vi "PH_BeamlineController.panel.vi"() -> ()   [LabVIEW 2014, in "PH_BeamlineController.lvlib"]
uses:
  PH_BeamlineController.lvlib
  PH_Beamline_Chief/PH_Beamline_Chief.Section.ctl
  PH_BeamlineInformation/PH_BeamlineInformation.Powermeter.ctl
  PH_BeamlineInformation/PH_BeamlineInformation.Efficiency.ctl
  PH_SystemInformation/PH_SystemInformation.GUI Refs.ctl
  PH_BeamlineController.Source Attributes.ctl
  PH_BeamlineController.Sources.ctl
  PH_BeamlineController.Target Attributes.ctl
  PH_BeamlineController.Targets.ctl
  PH_BeamlineController.PA DP Target Attributes.ctl
  PH_BeamlineController.PA DP Targets.ctl
  PH_BeamlineController.special GUI Refs.ctl
  PH_BeamlineInformation/PH_BeamlineInformation.GUI Ref.ctl
  PH_Common/PH_Common.lvlib
  PH_Beamline_Chief/PH_Beamline_Chief.lvlib
  PH_BeamlineInformation/PH_BeamlineInformation.lvlib
  PH_Synchrolock_Watch/PH_Synchrolock_Watch.lvlib
  PH_BackreflectionMeas/PH_BackreflectionMeas.lvlib
  CSCore/CSSystem/CSSystemLib/CSSystemLib.lvlib
  PH_SystemInformation/PH_SystemInformation.lvlib
  PH_Class/PH_Class.lvlib
panel:
  in  "Accept":bool
  out "PIL_Exp4_ShutterDisabled":u32(colorbox)=6618880 caption="Z6 enabled"
  out "Emergency Off":u32(colorbox)=16711680
  out "Laser enabled":u32(colorbox)=6618880
  out "PHELIX_Beamline_MA_LB_BL_Status 2":u32(colorbox)
  in  "PA-Backreflection-Meas":bool caption="B"
  in  "fs_Synchrolock_Watch":bool caption="S"
  out "PHELIX_Beamline_PA_before_Bypass_BL_Status":u32(colorbox)
  out "PHELIX_Beamline_PA_BL_Status":u32(colorbox)
  out "PHELIX_Beamline_LB_TB2_BL_Status":u32(colorbox)
  out "PHELIX_Beamline_Z6_BL_Status":u32(colorbox)
  out "PHELIX_Beamline_LL_BL_Status":u32(colorbox)
  out "PHELIX_Beamline_MA_Exit_BL_Status":u32(colorbox)
  out "PHELIX_Beamline_PA_Exit_BL_Status":u32(colorbox)
  out "PHELIX_Beamline_PA_Input_BL_Status":u32(colorbox)
  out "PHELIX_Beamline_PA_UnDelay_BL_Status":u32(colorbox)
  out "PHELIX_Beamline_fs_YLF_BL_Status":u32(colorbox)
  out "PHELIX_Beamline_YLF_BL_Status 2":u32(colorbox)
  out "PHELIX_Beamline_ns_BL_Status 2":u32(colorbox)
  out "PHELIX_Beamline_PA_Bypass_BL_Status 3":u32(colorbox)
  out "PHELIX_Beamline_PA_Bypass_BL_Status 2":u32(colorbox)
  out "PHELIX_Beamline_PA_Bypass_BL_Status 1":u32(colorbox)
  out "PHELIX_Beamline_PA_Delay_BL_Status 3":u32(colorbox)
  out "PHELIX_Beamline_PA_Input_BL_Status 1":u32(colorbox)
  out "PHELIX_Beamline_PA_Delay_BL_Status 2":u32(colorbox)
  out "PHELIX_Beamline_MA_Z6_BL_Status":u32(colorbox)
  out "PHELIX_Beamline_MA_LB_BL_Status 1":u32(colorbox)
  out "PHELIX_Beamline_MA_LB_BL_Status":u32(colorbox)
  out "PHELIX_Beamline_YLF_BL_Status 1":u32(colorbox)
  out "PHELIX_Beamline_fs_BL_Status":u32(colorbox)
  out "PHELIX_Beamline_ns_BL_Status 1":u32(colorbox)
  out "PHELIX_Beamline_PA_LL_BL_Status 2":u32(colorbox)
  out "PHELIX_Beamline_PA_LL_BL_Status 1":u32(colorbox)
  out "PHELIX_Beamline_PA_MA_BL_Status":u32(colorbox)
  in  "Delete":bool
  out "error out":errorcluster
  in  "error in (no error)":errorcluster
  in  "object ref":refnum<vi>
  out "PHELIX_Beamline_LB_TB3_BL_Status":u32(colorbox)
  in  "Experiment Z6":bool caption="Z6"
  in  "Experiment Laserlabor":bool caption="LL"
  in  "Calorimeter":bool caption="MA"
  in  "PreAmp":bool caption="PA"
  in  "ns-Frontend":bool caption="ns"
  in  "fs-Frontend":bool caption="fs"
  in  "YLF":bool
  in  "Dump Laserbay":bool
  in  "Dump Z6":bool
  in  "Dump Laserlabor":bool
  in  "Dump PA Undelayed":bool
  in  "Dump PA Delayed":bool
  out "Experiment_VacuumControl_Experiment":bool caption="V"
  in  "Experiment Laserbay":bool caption="LB"
  # "PCS"
  # "3.40"
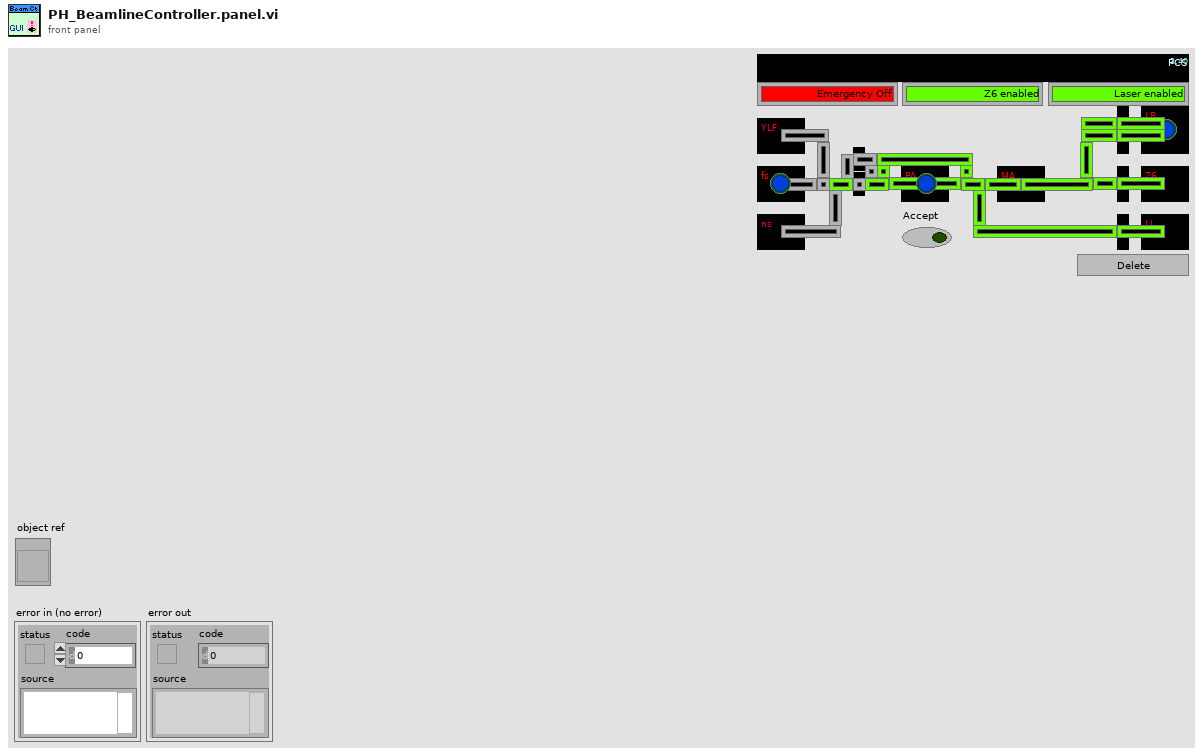
[diagram p1: front panel]
types:
  T1 = typedef "PH_BeamlineController.lvlib/PH_BeamlineController.Source Attributes.ctl" = cluster{"Name":T2, "GUI Ref":refnum<vi>, "Current State":bool, "Wanted State":bool}
  T2 = typedef "PH_BeamlineController.lvlib/PH_BeamlineController.Sources.ctl" = enum16{"None", "YLF", "fs-Frontend", "ns-Frontend", "YLF and ns-Frontend", "fs- and ns-Frontend"}
  T3 = typedef "PH_BeamlineController.lvlib/PH_BeamlineController.PA DP Target Attributes.ctl" = cluster{"Name":T4, "GUI Ref":refnum<vi>, "Current State":bool, "Wanted State":bool, "Enabled":bool}
  T4 = typedef "PH_BeamlineController.lvlib/PH_BeamlineController.PA DP Targets.ctl" = enum16{"None", "Dump PA Delayed Beam", "Dump PA Undelayed Beam", "Dumps PA Delayed and Undelayed Beam"}
  T5 = typedef "PH_BeamlineController.lvlib/PH_BeamlineController.Target Attributes.ctl" = cluster{"Name":T6, "GUI Ref":refnum<vi>, "Current State":bool, "Wanted State":bool, "Enabled":bool}
  T6 = typedef "PH_BeamlineController.lvlib/PH_BeamlineController.Targets.ctl" = enum16{"None", "PreAmp", "Dump Exp Laserlab", "Exp Laserlab", "Calorimeter", "Dump Exp Laserbay", "Exp Laserbay", "Dump Exp Z6", "Exp Z6"}
  T7 = typedef "PH_BeamlineController.lvlib/PH_BeamlineController.special GUI Refs.ctl" = cluster{"PA-Backreflection-Meas":refnum<vi>, "fs_Synchrolock_Watch":refnum<vi>}
  T8 = typedef "PH_BeamlineInformation.lvlib/PH_BeamlineInformation.GUI Ref.ctl" = cluster{"BL Elements":cluster{"GUI Ref":refnum<vi>, "Beamline Section":T9}[], "Powermeters":T10, "Efficiency GUI Refs":T11, "Head GUI Refs":cluster{"PA - 19 - 1":cluster{"in Use":refnum<vi>, "voltage":refnum<vi>}, "PA - 19 - 2":cluster{"in Use":refnum<vi>, "voltage":refnum<vi>}, "PA - 45":cluster{"in Use":refnum<vi>, "voltage":refnum<vi>}, "PA - 45 - DP":cluster{"in Use":refnum<vi>, "voltage":refnum<vi>}, "MA - 1":cluster{"in Use":refnum<vi>, "voltage":refnum<vi>}, "MA - 2":cluster{"in Use":refnum<vi>, "voltage":refnum<vi>}, "MA - 3":cluster{"in Use":refnum<vi>, "voltage":refnum<vi>}, "MA - 4":cluster{"in Use":refnum<vi>, "voltage":refnum<vi>}, "MA - 5":cluster{"in Use":refnum<vi>, "voltage":refnum<vi>}, "MA - FR":cluster{"in Use":refnum<vi>, "voltage":refnum<vi>}}, "System Information GUI Refs":T12}
  T9 = typedef "PH_Beamline_Chief.lvlib/PH_Beamline_Chief.Section.ctl" = enum16{"None", "YLF", "fs", "fs-YLF", "ns", "PA-Input", "PA-Undelay", "PA-Delay", "PA-before-Bypass", "PA", "PA-Bypass", "PA-Exit", "PA-LL", "LL", "PA-MA", "MA-Exit", "MA-Z6", "Z6", "MA-LB", "LB-TB2", "LB-TB3"}
  T10 = typedef "PH_BeamlineInformation.lvlib/PH_BeamlineInformation.Powermeter.ctl" = cluster{"ns FE":cluster{"GUI Ref":refnum<vi>, "Value":dbl}, "fs FE":cluster{"GUI Ref":refnum<vi>, "Value":dbl}, "PA":cluster{"GUI Ref":refnum<vi>, "Value":dbl}, "MA":cluster{"GUI Ref":refnum<vi>, "Value":dbl}, "Z6 green":cluster{"GUI Ref":refnum<vi>, "Value":dbl}, "Z6 IR":cluster{"GUI Ref":refnum<vi>, "Value":dbl}, "Z6 COS":cluster{"GUI Ref":refnum<vi>, "Value":dbl}}
  T11 = typedef "PH_BeamlineInformation.lvlib/PH_BeamlineInformation.Efficiency.ctl" = cluster{"PA Gain":cluster{"GUI Ref":refnum<vi>, "Value":dbl}, "MA Gain":cluster{"GUI Ref":refnum<vi>, "Value":dbl}, "Z6 green Conversion":cluster{"GUI Ref":refnum<vi>, "Value":dbl}, "Z6 Comp Losses":cluster{"GUI Ref":refnum<vi>, "Value":dbl}}
  T12 = typedef "PH_SystemInformation.lvlib/PH_SystemInformation.GUI Refs.ctl" = cluster{"Laser":refnum<vi>, "PreAmp":refnum<vi>, "MainAmp":refnum<vi>, "Emergency Off":refnum<vi>, "Exp 1":refnum<vi>, "Exp 2":refnum<vi>, "Exp 3":refnum<vi>, "Exp 4":refnum<vi>, "Timing Mode GUI Ref":refnum<vi>}
  T13 = cluster{"Sources":T1[], "Side Targets":T3[], "Targets":T5[], "Experiment_VacuumControl_Experiment":refnum<vi>, "special GUI Refs":T7, "Beamline Information GUI Refs":T8}
  T14 = cluster{"PA - 19 - 1":cluster{"in Use":refnum<vi>, "voltage":refnum<vi>}, "PA - 19 - 2":cluster{"in Use":refnum<vi>, "voltage":refnum<vi>}, "PA - 45":cluster{"in Use":refnum<vi>, "voltage":refnum<vi>}, "PA - 45 - DP":cluster{"in Use":refnum<vi>, "voltage":refnum<vi>}, "MA - 1":cluster{"in Use":refnum<vi>, "voltage":refnum<vi>}, "MA - 2":cluster{"in Use":refnum<vi>, "voltage":refnum<vi>}, "MA - 3":cluster{"in Use":refnum<vi>, "voltage":refnum<vi>}, "MA - 4":cluster{"in Use":refnum<vi>, "voltage":refnum<vi>}, "MA - 5":cluster{"in Use":refnum<vi>, "voltage":refnum<vi>}, "MA - FR":cluster{"in Use":refnum<vi>, "voltage":refnum<vi>}}
  T15 = cluster{"GUI Ref":refnum<vi>, "Beamline Section":T9}
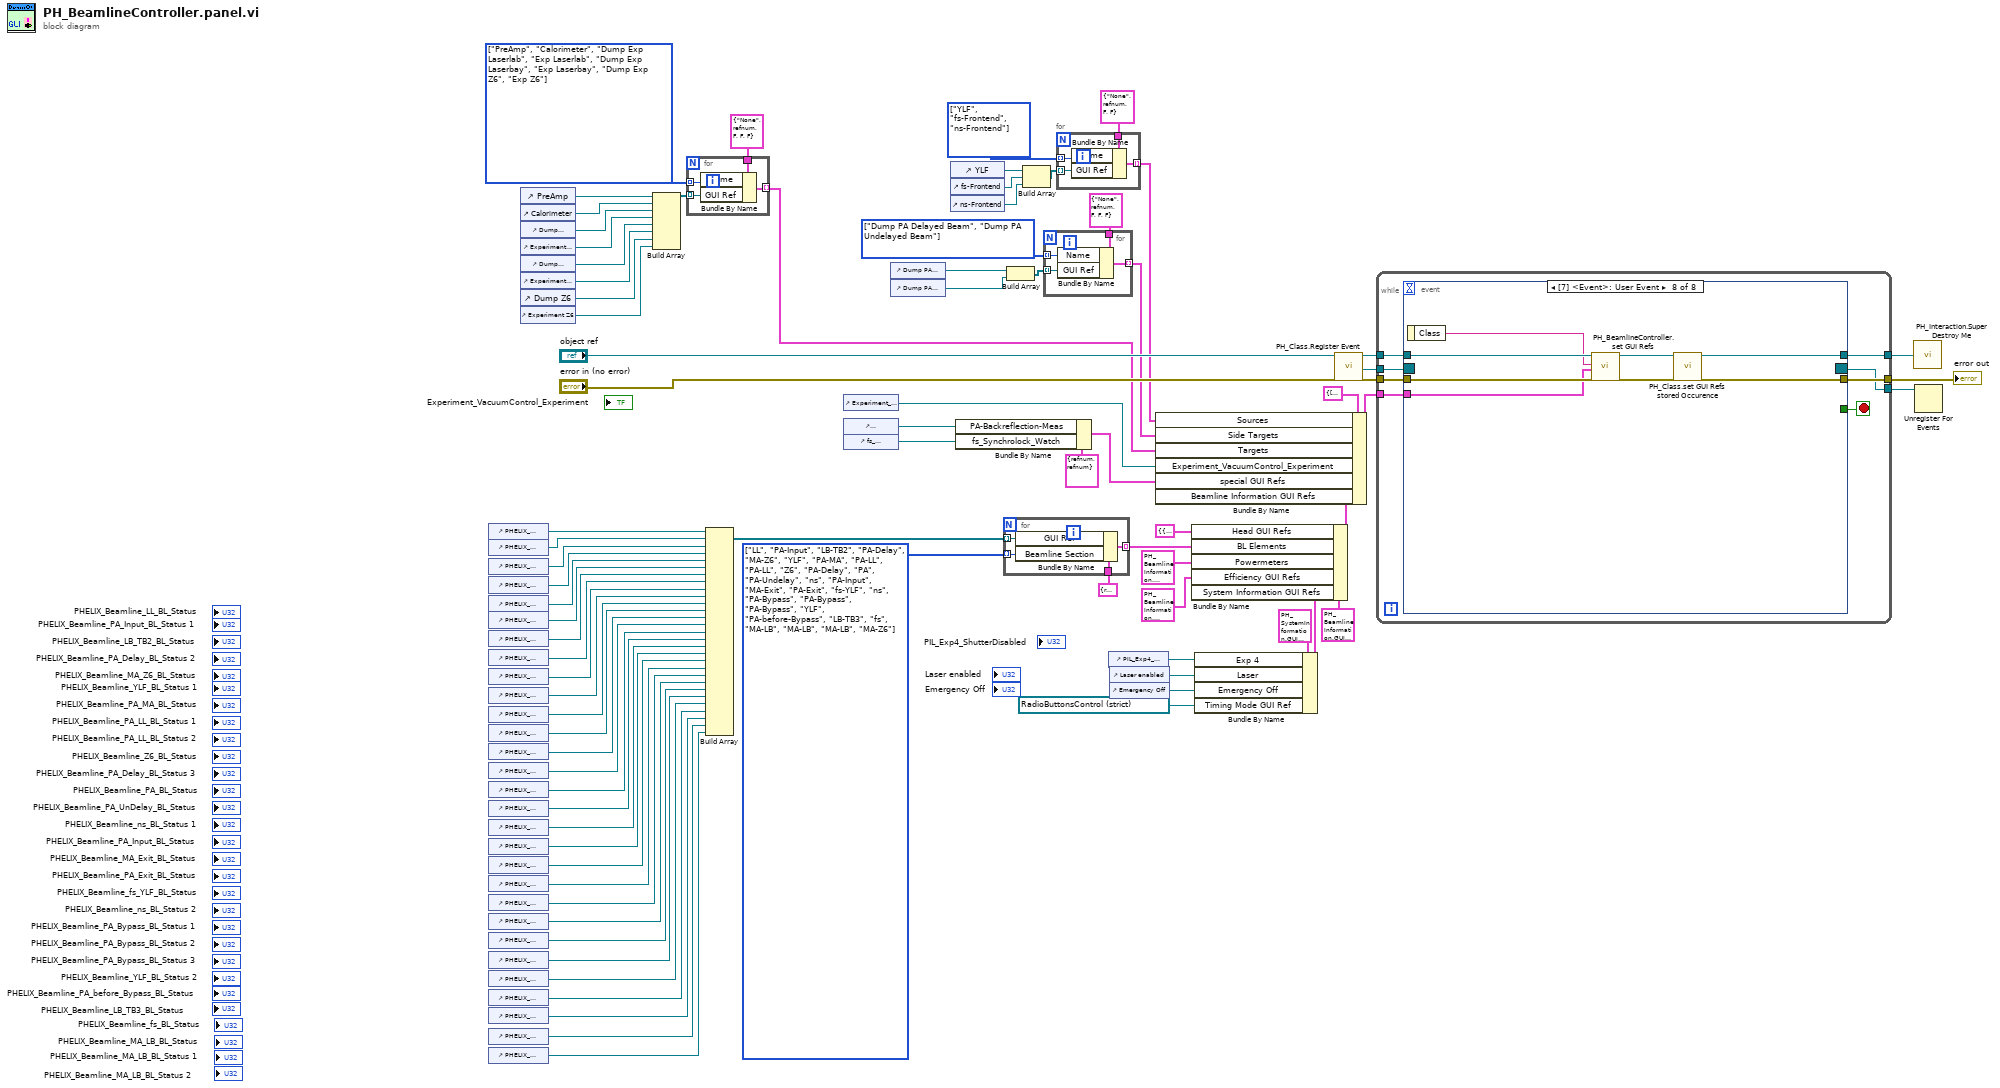
[diagram p0: block diagram]
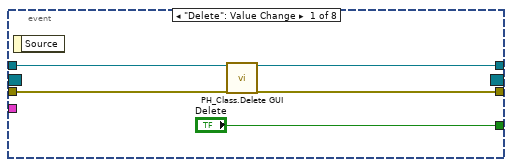
[diagram p2: hidden frame]
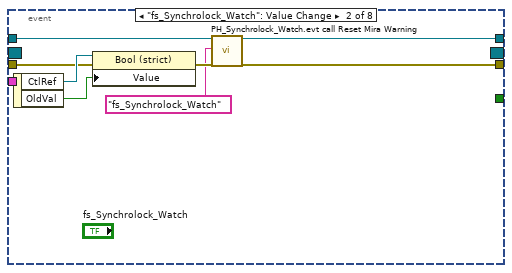
[diagram p3: hidden frame]
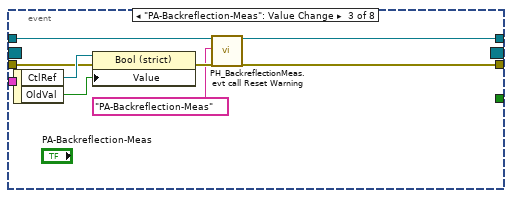
[diagram p4: hidden frame]
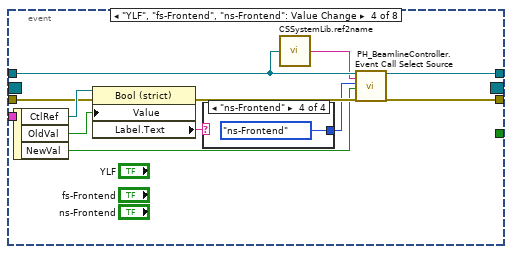
[diagram p5: hidden frame]
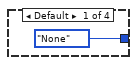
[diagram p6: hidden frame]
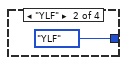
[diagram p7: hidden frame]
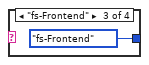
[diagram p8: hidden frame]
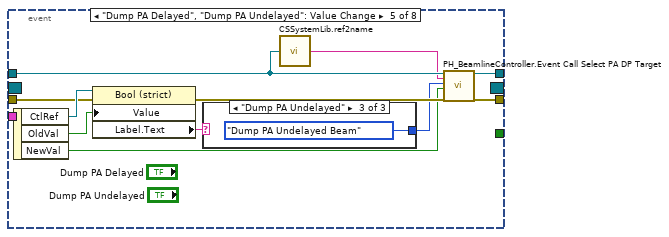
[diagram p9: hidden frame]
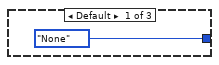
[diagram p10: hidden frame]
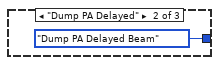
[diagram p11: hidden frame]
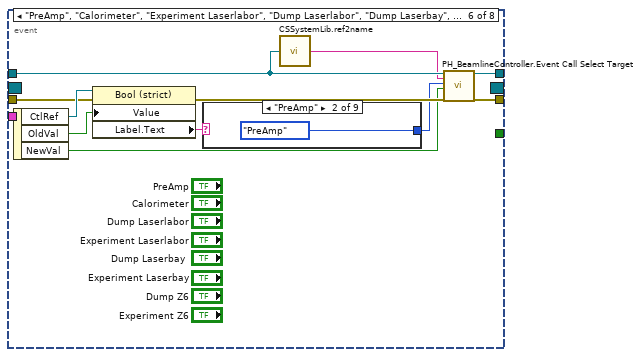
[diagram p12: hidden frame]
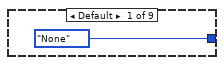
[diagram p13: hidden frame]
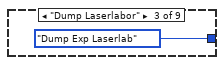
[diagram p14: hidden frame]
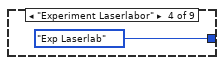
[diagram p15: hidden frame]
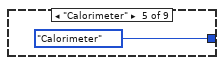
[diagram p16: hidden frame]
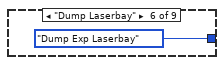
[diagram p17: hidden frame]
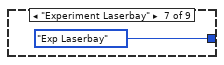
[diagram p18: hidden frame]
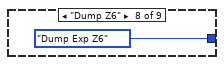
[diagram p19: hidden frame]
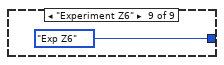
[diagram p20: hidden frame]
diagram:
  w17 = T4[] [enum."Dump PA Delayed Beam", enum."Dump PA Undelayed Beam"] items=["None", "Dump PA Delayed Beam", "Dump PA Undelayed Beam", "Dumps PA Delayed and Undelayed Beam"]
  w26 = T6[] [enum."PreAmp", enum."Calorimeter", enum."Dump Exp Laserlab", enum."Exp Laserlab", enum."Dump Exp Laserbay", enum."Exp Laserbay", enum."Dump Exp Z6", enum."Exp Z6"] items=["None", "PreAmp", "Dump Exp Laserlab", "Exp Laserlab", "Calorimeter", "Dump Exp Laserbay", "Exp Laserbay", "Dump Exp Z6", "Exp Z6"]
  w41 = T2[] [enum."YLF", enum."fs-Frontend", enum."ns-Frontend"] items=["None", "YLF", "fs-Frontend", "ns-Frontend", "YLF and ns-Frontend", "fs- and ns-Frontend"]
  w51 = T9[] [enum."LL", enum."PA-Input", enum."LB-TB2", enum."PA-Delay", enum."MA-Z6", enum."YLF", enum."PA-MA", enum."PA-LL", enum."PA-LL", enum."Z6", enum."PA-Delay", enum."PA", enum."PA-Undelay", enum."ns", enum."PA-Input", enum."MA-Exit", enum."PA-Exit", enum."fs-YLF", enum."ns", enum."PA-Bypass", enum."PA-Bypass", enum."PA-Bypass", enum."YLF", enum."PA-before-Bypass", enum."LB-TB3", enum."fs", enum."MA-LB", enum."MA-LB", enum."MA-LB", enum."MA-Z6"] items=["None", "YLF", "fs", "fs-YLF", "ns", "PA-Input", "PA-Undelay", "PA-Delay", "PA-before-Bypass", "PA", "PA-Bypass", "PA-Exit", "PA-LL", "LL", "PA-MA", "MA-Exit", "MA-Z6", "Z6", "MA-LB", "LB-TB2", "LB-TB3"]
  n1 = control-ref of="PHELIX_Beamline_LL_BL_Status"() -> (w82:refnum<vi>)
  n2 = control-ref of="PHELIX_Beamline_PA_Input_BL_Status 1"() -> (w81:refnum<vi>)
  n3 = control-ref of="PHELIX_Beamline_LB_TB2_BL_Status"() -> (w80:refnum<vi>)
  n4 = control-ref of="PHELIX_Beamline_PA_Delay_BL_Status 2"() -> (w79:refnum<vi>)
  n5 = control-ref of="PHELIX_Beamline_MA_Z6_BL_Status"() -> (w78:refnum<vi>)
  n6 = control-ref of="PHELIX_Beamline_YLF_BL_Status 1"() -> (w77:refnum<vi>)
  n7 = control-ref of="PHELIX_Beamline_PA_MA_BL_Status"() -> (w76:refnum<vi>)
  n8 = control-ref of="PHELIX_Beamline_PA_LL_BL_Status 1"() -> (w75:refnum<vi>)
  n9 = control-ref of="PHELIX_Beamline_PA_LL_BL_Status 2"() -> (w74:refnum<vi>)
  n10 = control-ref of="PHELIX_Beamline_Z6_BL_Status"() -> (w73:refnum<vi>)
  n11 = control-ref of="PHELIX_Beamline_PA_Delay_BL_Status 3"() -> (w72:refnum<vi>)
  n12 = control-ref of="PHELIX_Beamline_PA_BL_Status"() -> (w71:refnum<vi>)
  n13 = control-ref of="PHELIX_Beamline_PA_UnDelay_BL_Status"() -> (w70:refnum<vi>)
  n14 = control-ref of="PHELIX_Beamline_ns_BL_Status 1"() -> (w69:refnum<vi>)
  n15 = control-ref of="PHELIX_Beamline_PA_Input_BL_Status"() -> (w68:refnum<vi>)
  n16 = control-ref of="PHELIX_Beamline_MA_Exit_BL_Status"() -> (w67:refnum<vi>)
  n17 = control-ref of="PHELIX_Beamline_PA_Exit_BL_Status"() -> (w66:refnum<vi>)
  n18 = control-ref of="PHELIX_Beamline_fs_YLF_BL_Status"() -> (w65:refnum<vi>)
  n19 = control-ref of="PHELIX_Beamline_ns_BL_Status 2"() -> (w64:refnum<vi>)
  n20 = control-ref of="PHELIX_Beamline_PA_Bypass_BL_Status 1"() -> (w63:refnum<vi>)
  n21 = control-ref of="PHELIX_Beamline_PA_Bypass_BL_Status 2"() -> (w62:refnum<vi>)
  n22 = control-ref of="PHELIX_Beamline_PA_Bypass_BL_Status 3"() -> (w61:refnum<vi>)
  n23 = control-ref of="PHELIX_Beamline_YLF_BL_Status 2"() -> (w60:refnum<vi>)
  n24 = control-ref of="PHELIX_Beamline_PA_before_Bypass_BL_Status"() -> (w59:refnum<vi>)
  n25 = control-ref of="PHELIX_Beamline_LB_TB3_BL_Status"() -> (w58:refnum<vi>)
  n26 = control-ref of="PHELIX_Beamline_fs_BL_Status"() -> (w57:refnum<vi>)
  n27 = control-ref of="PHELIX_Beamline_MA_LB_BL_Status"() -> (w56:refnum<vi>)
  n28 = control-ref of="PHELIX_Beamline_MA_LB_BL_Status 1"() -> (w55:refnum<vi>)
  n29 = control-ref of="PHELIX_Beamline_MA_LB_BL_Status 2"() -> (w54:refnum<vi>)
  n30 = control-ref of="PreAmp"() -> (w35:refnum<vi>)
  n31 = control-ref of="Calorimeter"() -> (w34:refnum<vi>)
  n32 = control-ref of="Dump Laserlabor"() -> (w33:refnum<vi>)
  n33 = control-ref of="Experiment Laserlabor"() -> (w32:refnum<vi>)
  n34 = control-ref of="Dump Laserbay"() -> (w31:refnum<vi>)
  n35 = control-ref of="Experiment Laserbay"() -> (w30:refnum<vi>)
  n36 = control-ref of="Dump Z6"() -> (w29:refnum<vi>)
  n37 = control-ref of="Experiment Z6"() -> (w28:refnum<vi>)
  n38 = Build Array(w35, w34, w33, w32, w31, w30, w29, w28) -> (w27:refnum<vi>[])
  n39 = for {
    tunnel: T5 {"Name"=enum."None", "GUI Ref"=refnum, "Current State"=FALSE, "Wanted State"=FALSE, "Enabled"=FALSE} ("Target Attributes") -> [w88]
    tunnel: [w87] -> w1 mode=indexing
    tunnel: w26 -> [w86] mode=indexing
    tunnel: w27 -> [w85] mode=indexing
    n40 = Bundle By Name(cluster=w88, "Name"=w86, "GUI Ref"=w85) -> (w87:T5)
  }
  n41 = Build Array(w82, w81, w80, w79, w78, w77, w76, w75, w74, w73, w72, w71, w70, w69, w68, w67, w66, w65, w64, w63, w62, w61, w60, w59, w58, w57, w56, w55, w54) -> (w52:refnum<vi>[])
  n42 = control-ref of="Experiment_VacuumControl_Experiment"() -> (w5:refnum<vi>)
  n43 = control-ref of="PA-Backreflection-Meas"() -> (w20:refnum<vi>)
  n44 = control-ref of="fs_Synchrolock_Watch"() -> (w19:refnum<vi>)
  n45 = control-ref of="Dump PA Delayed"() -> (w24:refnum<vi>)
  n46 = control-ref of="Dump PA Undelayed"() -> (w18:refnum<vi>)
  n47 = control-ref of="YLF"() -> (w40:refnum<vi>)
  n48 = control-ref of="fs-Frontend"() -> (w39:refnum<vi>)
  n49 = control-ref of="ns-Frontend"() -> (w38:refnum<vi>)
  n50 = Bundle By Name(cluster=T7 {"PA-Backreflection-Meas"=refnum, "fs_Synchrolock_Watch"=refnum} ("GUI Refs"), "PA-Backreflection-Meas"=w20, "fs_Synchrolock_Watch"=w19) -> (w4:T7)
  n51 = for {
    tunnel: T15 {"GUI Ref"=refnum, "Beamline Section"=enum."None"} ("BL Element") -> [w92]
    tunnel: [w91] -> w48 mode=indexing
    tunnel: w52 -> [w90] mode=indexing
    tunnel: w51 -> [w89] mode=indexing
    n52 = Bundle By Name(cluster=w92, "GUI Ref"=w90, "Beamline Section"=w89) -> (w91:T15)
  }
  n53 = Build Array(w24, w18) -> (w23:refnum<vi>[])
  n54 = Build Array(w40, w39, w38) -> (w37:refnum<vi>[])
  n55 = for {
    tunnel: T3 {"Name"=enum."None", "GUI Ref"=refnum, "Current State"=FALSE, "Wanted State"=FALSE, "Enabled"=FALSE} ("Target") -> [w96]
    tunnel: [w95] -> w6 mode=indexing
    tunnel: w17 -> [w94] mode=indexing
    tunnel: w23 -> [w93] mode=indexing
    n56 = Bundle By Name(cluster=w96, "Name"=w94, "GUI Ref"=w93) -> (w95:T3)
  }
  n57 = for {
    tunnel: T1 {"Name"=enum."None", "GUI Ref"=refnum, "Current State"=FALSE, "Wanted State"=FALSE} ("Source Attributes") -> [w100]
    tunnel: [w99] -> w7 mode=indexing
    tunnel: w41 -> [w98] mode=indexing
    tunnel: w37 -> [w97] mode=indexing
    n58 = Bundle By Name(cluster=w100, "Name"=w98, "GUI Ref"=w97) -> (w99:T1)
  }
  n59 = control-ref of="PIL_Exp4_ShutterDisabled"() -> (w22:refnum<vi>)
  n60 = control-ref of="Laser enabled"() -> (w44:refnum<vi>)
  n61 = control-ref of="Emergency Off"() -> (w43:refnum<vi>)
  n62 = Bundle By Name(cluster=T12 {"Laser"=refnum, "PreAmp"=refnum, "MainAmp"=refnum, "Emergency Off"=refnum, "Exp 1"=refnum, "Exp 2"=refnum, "Exp 3"=refnum, "Exp 4"=refnum, "Timing Mode GUI Ref"=refnum} ("Input for System Information"), "Exp 4"=w22, "Laser"=w44, "Emergency Off"=w43, "Timing Mode GUI Ref"=refnum<vi> refnum) -> (w15:T12)
  n63 = Bundle By Name(cluster=T8 {"BL Elements"=[], "Powermeters"={"ns FE"={"GUI Ref"=refnum, "Value"=-1.0}, "fs FE"={"GUI Ref"=refnum, "Value"=-1.0}, "PA"={"GUI Ref"=refnum, "Value"=-1.0}, "MA"={"GUI Ref"=refnum, "Value"=-1.0}, "Z6 green"={"GUI Ref"=refnum, "Value"=-1.0}, "Z6 IR"={"GUI Ref"=refnum, "Value"=-1.0}, "Z6 COS"={"GUI Ref"=refnum, "Value"=-1.0}}, "Efficiency GUI Refs"={"PA Gain"={"GUI Ref"=refnum, "Value"=-1.0}, "MA Gain"={"GUI Ref"=refnum, "Value"=-1.0}, "Z6 green Conversion"={"GUI Ref"=refnum, "Value"=-1.0}, "Z6 Comp Losses"={"GUI Ref"=refnum, "Value"=-1.0}}, "Head GUI Refs"={"PA - 19 - 1"={"in Use"=refnum, "voltage"=refnum}, "PA - 19 - 2"={"in Use"=refnum, "voltage"=refnum}, "PA - 45"={"in Use"=refnum, "voltage"=refnum}, "PA - 45 - DP"={"in Use"=refnum, "voltage"=refnum}, "MA - 1"={"in Use"=refnum, "voltage"=refnum}, "MA - 2"={"in Use"=refnum, "voltage"=refnum}, "MA - 3"={"in Use"=refnum, "voltage"=refnum}, "MA - 4"={"in Use"=refnum, "voltage"=refnum}, "MA - 5"={"in Use"=refnum, "voltage"=refnum}, "MA - FR"={"in Use"=refnum, "voltage"=refnum}}, "System Information GUI Refs"={"Laser"=refnum, "PreAmp"=refnum, "MainAmp"=refnum, "Emergency Off"=refnum, "Exp 1"=refnum, "Exp 2"=refnum, "Exp 3"=refnum, "Exp 4"=refnum, "Timing Mode GUI Ref"=refnum}} ("BeamlineInformation GUI Refs"), "Head GUI Refs"=T14 {"PA - 19 - 1"={"in Use"=refnum, "voltage"=refnum}, "PA - 19 - 2"={"in Use"=refnum, "voltage"=refnum}, "PA - 45"={"in Use"=refnum, "voltage"=refnum}, "PA - 45 - DP"={"in Use"=refnum, "voltage"=refnum}, "MA - 1"={"in Use"=refnum, "voltage"=refnum}, "MA - 2"={"in Use"=refnum, "voltage"=refnum}, "MA - 3"={"in Use"=refnum, "voltage"=refnum}, "MA - 4"={"in Use"=refnum, "voltage"=refnum}, "MA - 5"={"in Use"=refnum, "voltage"=refnum}, "MA - FR"={"in Use"=refnum, "voltage"=refnum}}, "BL Elements"=w48, "Powermeters"=T10 {"ns FE"={"GUI Ref"=refnum, "Value"=-1.0}, "fs FE"={"GUI Ref"=refnum, "Value"=-1.0}, "PA"={"GUI Ref"=refnum, "Value"=-1.0}, "MA"={"GUI Ref"=refnum, "Value"=-1.0}, "Z6 green"={"GUI Ref"=refnum, "Value"=-1.0}, "Z6 IR"={"GUI Ref"=refnum, "Value"=-1.0}, "Z6 COS"={"GUI Ref"=refnum, "Value"=-1.0}}, "Efficiency GUI Refs"=T11 {"PA Gain"={"GUI Ref"=refnum, "Value"=-1.0}, "MA Gain"={"GUI Ref"=refnum, "Value"=-1.0}, "Z6 green Conversion"={"GUI Ref"=refnum, "Value"=-1.0}, "Z6 Comp Losses"={"GUI Ref"=refnum, "Value"=-1.0}}, "System Information GUI Refs"=w15) -> (w3:T8)
  n64 = Bundle By Name(cluster=T13 {"Sources"=[], "Side Targets"=[], "Targets"=[], "Experiment_VacuumControl_Experiment"=refnum, "special GUI Refs"={"PA-Backreflection-Meas"=refnum, "fs_Synchrolock_Watch"=refnum}, "Beamline Information GUI Refs"={"BL Elements"=[], "Powermeters"={"ns FE"={"GUI Ref"=refnum, "Value"=-1.0}, "fs FE"={"GUI Ref"=refnum, "Value"=-1.0}, "PA"={"GUI Ref"=refnum, "Value"=-1.0}, "MA"={"GUI Ref"=refnum, "Value"=-1.0}, "Z6 green"={"GUI Ref"=refnum, "Value"=-1.0}, "Z6 IR"={"GUI Ref"=refnum, "Value"=-1.0}, "Z6 COS"={"GUI Ref"=refnum, "Value"=-1.0}}, "Efficiency GUI Refs"={"PA Gain"={"GUI Ref"=refnum, "Value"=-1.0}, "MA Gain"={"GUI Ref"=refnum, "Value"=-1.0}, "Z6 green Conversion"={"GUI Ref"=refnum, "Value"=-1.0}, "Z6 Comp Losses"={"GUI Ref"=refnum, "Value"=-1.0}}, "Head GUI Refs"={"PA - 19 - 1"={"in Use"=refnum, "voltage"=refnum}, "PA - 19 - 2"={"in Use"=refnum, "voltage"=refnum}, "PA - 45"={"in Use"=refnum, "voltage"=refnum}, "PA - 45 - DP"={"in Use"=refnum, "voltage"=refnum}, "MA - 1"={"in Use"=refnum, "voltage"=refnum}, "MA - 2"={"in Use"=refnum, "voltage"=refnum}, "MA - 3"={"in Use"=refnum, "voltage"=refnum}, "MA - 4"={"in Use"=refnum, "voltage"=refnum}, "MA - 5"={"in Use"=refnum, "voltage"=refnum}, "MA - FR"={"in Use"=refnum, "voltage"=refnum}}, "System Information GUI Refs"={"Laser"=refnum, "PreAmp"=refnum, "MainAmp"=refnum, "Emergency Off"=refnum, "Exp 1"=refnum, "Exp 2"=refnum, "Exp 3"=refnum, "Exp 4"=refnum, "Timing Mode GUI Ref"=refnum}}} ("Beamline Controller GUI Refs"), "Sources"=w7, "Side Targets"=w6, "Targets"=w1, "Experiment_VacuumControl_Experiment"=w5, "special GUI Refs"=w4, "Beamline Information GUI Refs"=w3) -> (w2:T13)
  n65 = call "PH_Class.Register Event.vi"("i ref in"="object ref", "error in (no error)"="error in (no error)") -> ("i ref out"=w14:refnum<vi>, "Event Registration Refnum"=w12:refnum<event-registration>, "error out"=w13:errorcluster)  [unwired: 15 in]
  n66 = while {
    tunnel: w14 -> [w105]
    tunnel: [w104] -> w84
    tunnel: [w107] -> w83
    tunnel: w13 -> [w106]
    tunnel: w12 -> [w103]
    tunnel: [w102] -> w11
    tunnel: w2 -> [w101]
    stop <- w108 stop-if-true
    n67 = event shown="[7] <Event>: User Event" {
      selector: w103 -> [_ _ _ _ _ _ _ _]
      dyn-events: [_ _ _ _ _ _ _ _] -> w102
      timeout: _ -> [_ _ _ _ _ _ _ _]
      tunnel: ["Delete" _ _ _ _ _ _ _] -> w108
      tunnel: w105 -> [w110 w116 w124 w131 w146 w160 w181 w191]
      tunnel: [w112 w120 w128 w139 w154 w168 w182 w186] -> w107
      tunnel: w106 -> [w109 w115 w123 w135 w150 w164 w179 w190]
      tunnel: [w111 w121 w129 w140 w155 w169 w183 w184] -> w104
      tunnel: w101 -> [_ _ _ _ _ _ _ w187]
      event "Delete": Value Change {
        n68 = event-data() -> ()  [unwired: 1 in, 1 out]
        n69 = call "PH_Class.Delete GUI.vi"("VI in"=w110, "error in (no error)"=w109) -> ("VI out"=w111:refnum<vi>, "error out"=w112:errorcluster)  [unwired: 16 in]
      }
      event "fs_Synchrolock_Watch": Value Change {
        n70 = event-data() -> ("CtlRef"=w118:refnum<vi>, "OldVal"=w117:bool)  [unwired: 1 in]
        n71 = property class="Bool (strict)"(reference=w118, error in=w115, "Value"=w117) -> (error out=w119:errorcluster)  [unwired: 1 out]
        n72 = call "PH_Synchrolock_Watch.evt call Reset Mira Warning.vi"("i ref in"=w116, "Instance"="fs_Synchrolock_Watch" ("Synchrolock.Instance"), "error in (no error)"=w119) -> ("i ref out"=w121:refnum<vi>, "error out"=w120:errorcluster)  [unwired: 15 in]
      }
      event "PA-Backreflection-Meas": Value Change {
        n73 = event-data() -> ("CtlRef"=w126:refnum<vi>, "OldVal"=w125:bool)  [unwired: 1 in]
        n74 = property class="Bool (strict)"(reference=w126, error in=w123, "Value"=w125) -> (error out=w127:errorcluster)  [unwired: 1 out]
        n75 = call "PH_BackreflectionMeas.evt call Reset Warning.vi"("i ref in"=w124, "Instance"="PA-Backreflection-Meas" ("Instance PA Backreflection"), "error in (no error)"=w127) -> ("i ref out"=w129:refnum<vi>, "error out"=w128:errorcluster)  [unwired: 15 in]
      }
      event "YLF", "fs-Frontend", "ns-Frontend": Value Change {
        n76 = event-data() -> ("CtlRef"=w137:refnum<vi>, "OldVal"=w136:bool, "NewVal"=w133:bool)  [unwired: 1 in]
        n77 = property class="Bool (strict)"(reference=w137, error in=w135, "Value"=w136) -> (error out=w138:errorcluster, "Label.Text"=w132:string)  [unwired: 1 out]
        n78 = case shown="\"ns-Frontend\"" w132 {
          tunnel: [PH_BeamlineController.Sources."None" ("Source") PH_BeamlineController.Sources."YLF" ("Source") PH_BeamlineController.Sources."fs-Frontend" ("Source") PH_BeamlineController.Sources."ns-Frontend" ("Source")] -> w134
          frame Default {
          }
          frame "YLF" {
          }
          frame "fs-Frontend" {
          }
          frame "ns-Frontend" {
          }
        }
        n79 = call "CSSystemLib.ref2name.vi"("obj refnum"=w131) -> ("name"=w130:string)
        n80 = call "PH_BeamlineController.Event Call Select Source.vi"("i ref in"=w131, "Instance"=w130, "Source"=w134, "on(off"=w133, "error in (no error)"=w138) -> ("i ref out"=w140:refnum<vi>, "error out"=w139:errorcluster)  [unwired: 13 in]
      }
      event "Dump PA Delayed", "Dump PA Undelayed": Value Change {
        n81 = event-data() -> ("CtlRef"=w152:refnum<vi>, "OldVal"=w151:bool, "NewVal"=w148:bool)  [unwired: 1 in]
        n82 = property class="Bool (strict)"(reference=w152, error in=w150, "Value"=w151) -> (error out=w153:errorcluster, "Label.Text"=w147:string)  [unwired: 1 out]
        n83 = case shown="\"Dump PA Undelayed\"" w147 {
          tunnel: [PH_BeamlineController.PA_DP_Targets."None" ("Targets") PH_BeamlineController.PA_DP_Targets."Dump PA Delayed Beam" ("Targets") PH_BeamlineController.PA_DP_Targets."Dump PA Undelayed Beam" ("Targets")] -> w149
          frame Default {
          }
          frame "Dump PA Delayed" {
          }
          frame "Dump PA Undelayed" {
          }
        }
        n84 = call "CSSystemLib.ref2name.vi"("obj refnum"=w146) -> ("name"=w145:string)
        n85 = call "PH_BeamlineController.Event Call Select PA DP Target.vi"("i ref in"=w146, "Instance"=w145, "PA DP Targets"=w149, "on(off"=w148, "error in (no error)"=w153) -> ("i ref out"=w155:refnum<vi>, "error out"=w154:errorcluster)  [unwired: 13 in]
      }
      event "PreAmp", "Calorimeter", "Experiment Laserlabor", "Dump Laserlabor", "Dump Laserbay", "Experiment Laserbay", "Dump Z6", "Experiment Z6": Value Change {
        n86 = event-data() -> ("CtlRef"=w166:refnum<vi>, "OldVal"=w165:bool, "NewVal"=w162:bool)  [unwired: 1 in]
        n87 = property class="Bool (strict)"(reference=w166, error in=w164, "Value"=w165) -> (error out=w167:errorcluster, "Label.Text"=w161:string)  [unwired: 1 out]
        n88 = case shown="\"PreAmp\"" w161 {
          tunnel: [PH_BeamlineController.Targets."None" ("Targets") PH_BeamlineController.Targets."PreAmp" ("Targets") PH_BeamlineController.Targets."Dump Exp Laserlab" ("Targets") PH_BeamlineController.Targets."Exp Laserlab" ("Targets") PH_BeamlineController.Targets."Calorimeter" ("Targets") PH_BeamlineController.Targets."Dump Exp Laserbay" ("Targets") PH_BeamlineController.Targets."Exp Laserbay" ("Targets") PH_BeamlineController.Targets."Dump Exp Z6" ("Targets") PH_BeamlineController.Targets."Exp Z6" ("Targets")] -> w163
          frame Default {
          }
          frame "PreAmp" {
          }
          frame "Dump Laserlabor" {
          }
          frame "Experiment Laserlabor" {
          }
          frame "Calorimeter" {
          }
          frame "Dump Laserbay" {
          }
          frame "Experiment Laserbay" {
          }
          frame "Dump Z6" {
          }
          frame "Experiment Z6" {
          }
        }
        n89 = call "CSSystemLib.ref2name.vi"("obj refnum"=w160) -> ("name"=w159:string)
        n90 = call "PH_BeamlineController.Event Call Select Target.vi"("i ref in"=w160, "Instance"=w159, "Targets"=w163, "on(off"=w162, "error in (no error)"=w167) -> ("i ref out"=w169:refnum<vi>, "error out"=w168:errorcluster)  [unwired: 13 in]
      }
      event "Accept": Value Change {
        n91 = event-data() -> ()  [unwired: 1 in, 3 out]
        n92 = call "CSSystemLib.ref2name.vi"("obj refnum"=w181) -> ("name"=w180:string)
        n93 = call "PH_BeamlineController.Event Call Accept.vi"("i ref in"=w181, "Instance"=w180, "error in (no error)"=w179) -> ("i ref out"=w183:refnum<vi>, "error out"=w182:errorcluster)  [unwired: 15 in]
      }
      event User Event {
        n94 = event-data() -> ("Class"=w188:string)  [unwired: 1 in]
        n95 = call "PH_BeamlineController.set GUI Refs.vi"("Ref in"=w191, "Class"=w188, "Beamline Controller GUI Refs"=w187, "error in"=w190) -> ("Ref out"=w185:refnum<vi>, "error out"=w189:errorcluster)  [unwired: 14 in]
        n96 = call "PH_Class.set GUI Refs stored Occurence.vi"("i ref in"=w185, "error in (no error)"=w189) -> ("i ref out"=w184:refnum<vi>, "error out"=w186:errorcluster)  [unwired: 16 in]
      }
    }
  }
  "error out" <- w83
  n97 = call "PH_Interaction.Super Destroy Me.vi"("i ref out"=w84) -> ()
  n98 = Unregister For Events(event registration refnum=w11) -> ()  [unwired: 1 in, 1 out]
